vi "S2C_SaveScriptAs.vi"(8 "Error In":errorcluster) -> (0 "Error Out":errorcluster)   [LabVIEW 2015]
doc: "Prompts for file name, checks the script settings, and saves the script to a local file."
uses:
  Globals/S2C_Globals.vi
  <vilib>/Utility/config.llb/Write Key (String).vi
  <vilib>/Utility/config.llb/NI_LVConfig.lvlib
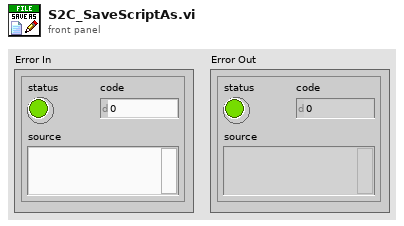
[diagram p1: front panel]
types:
  T1 = typedef "NI_LVConfig.lvlib/Config Data RefNum.ctl" = refnum<k1>
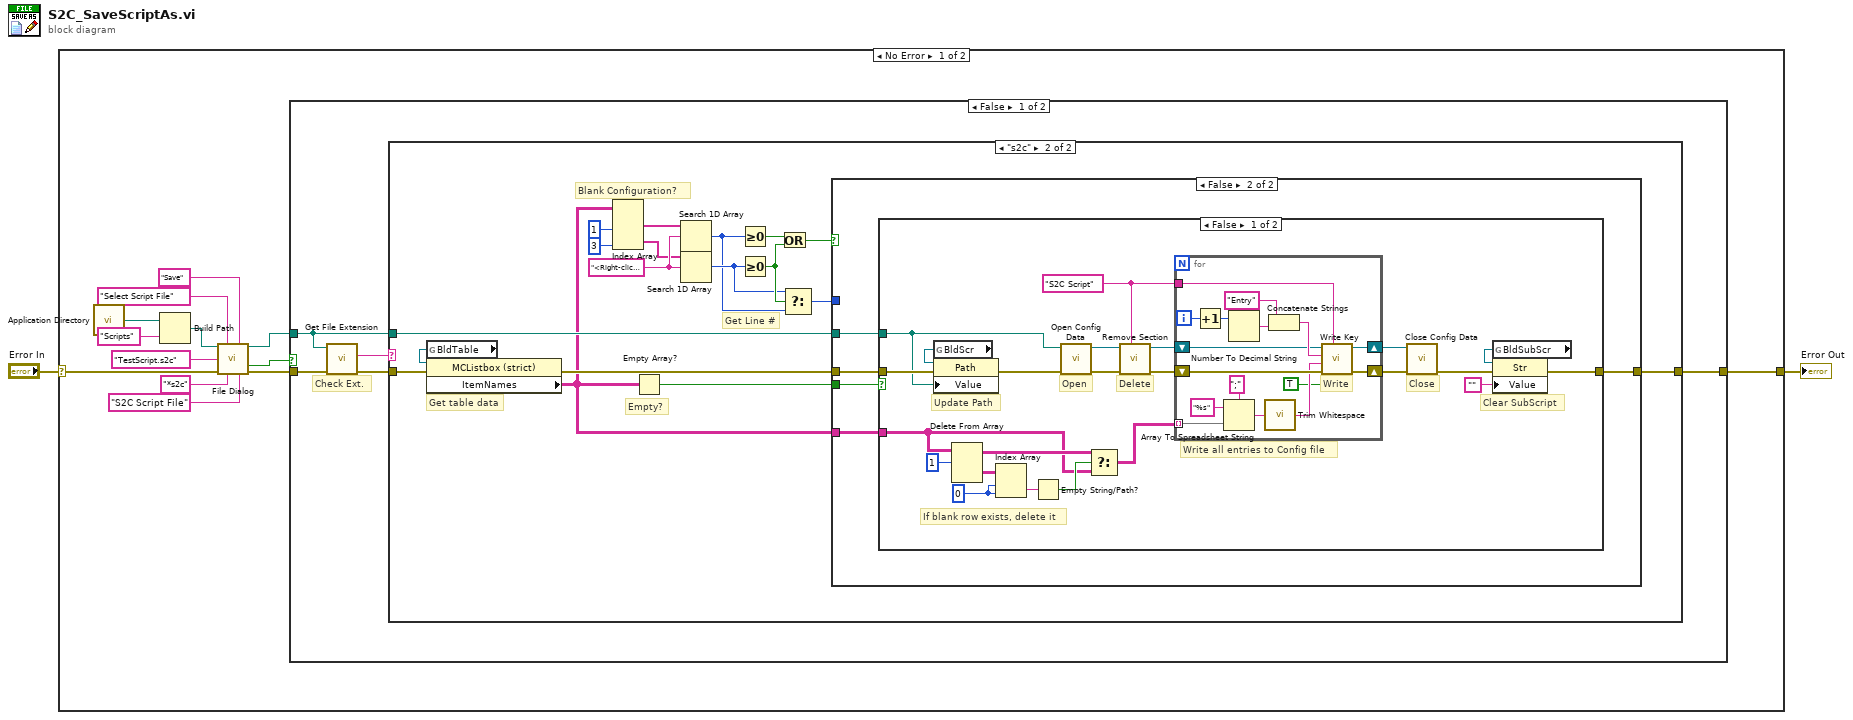
[diagram p0: block diagram]
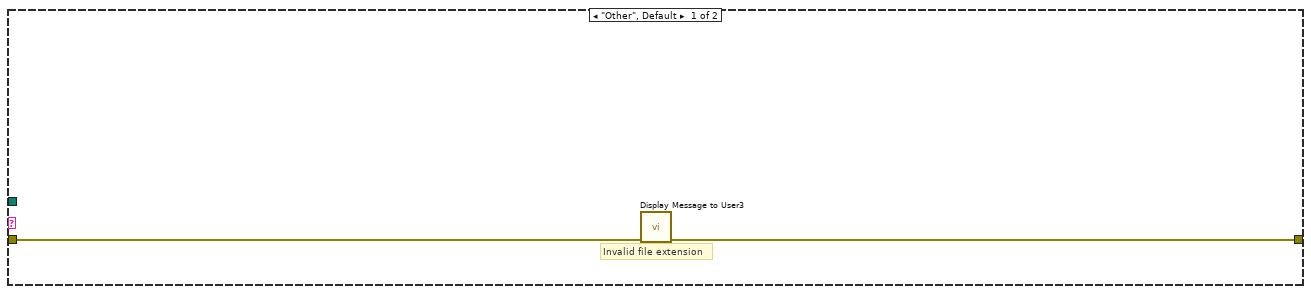
[diagram p2: hidden frame]
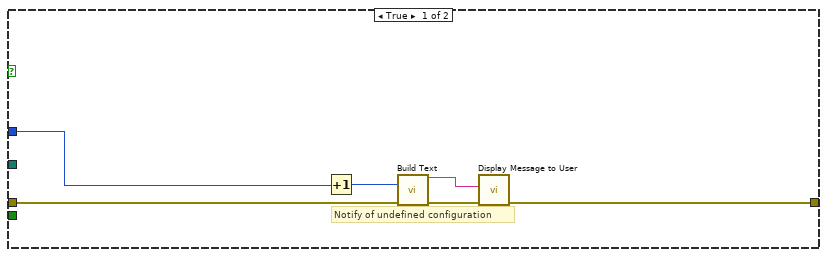
[diagram p3: hidden frame]
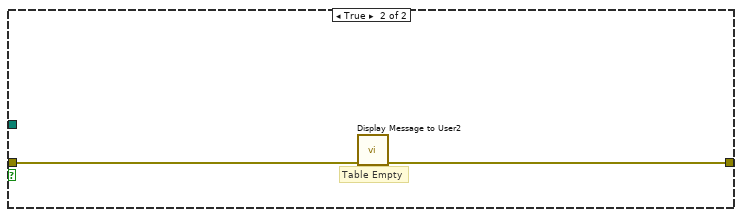
[diagram p4: hidden frame]
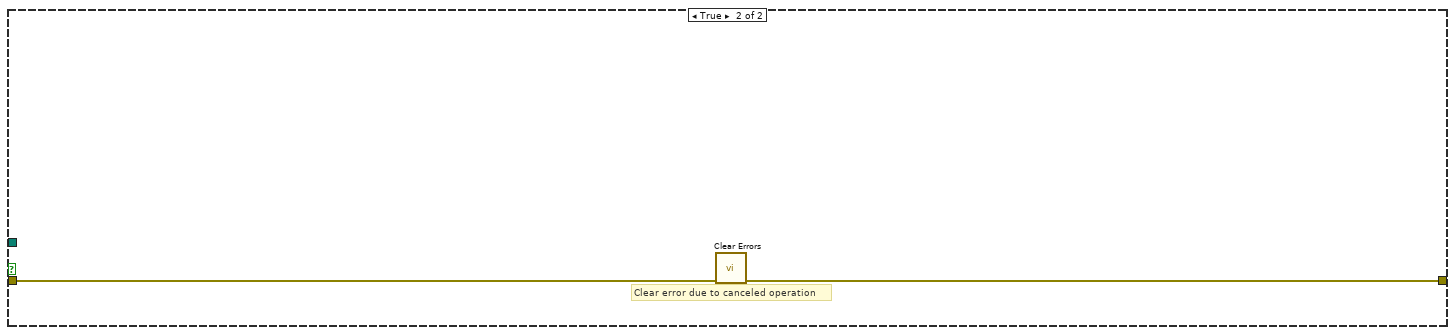
[diagram p5: hidden frame]
diagram:
  n1 = case shown="No Error" "Error In" {
    selector: "Error In" -> [w15 w95]
    tunnel: [w3 w95] -> w1
    frame No Error {
      n2 = call <vilib>:"Application Directory.vi"() -> ("Application Directory"=w13:path)
      n3 = Build Path(base path=w13, name or relative path="Scripts") -> (appended path=w11:path)
      n4 = call "File Dialog"("start path"=w11, "prompt"="Select Script File", "button label"="Save", "default name"="TestScript.s2c", "error in"=w15, "pattern (all files)"="*s2c", "pattern label"="S2C Script File") -> ("selected path"=w4:path, "cancelled"=w5:bool, "error out"=w6:errorcluster)  [unwired: 5 in, 1 out]
      n5 = case shown="False" w5 {
        tunnel: w6 -> [w19 w94]
        tunnel: w4 -> [w16 _]
        tunnel: [w20 w93] -> w3
        frame False {
          # "Check Ext."
          n6 = call <vilib>:"Get File Extension.vi"("error in (no error)"=w19, "file"=w16) -> ("error out"=w18:errorcluster, "lowercase file extension"=w17:string)  [unwired: 5 in, 3 out]
          n7 = case shown="\"s2c\"" w17 {
            tunnel: [w21 w39] -> w20
            tunnel: w18 -> [w22 w37]
            tunnel: w16 -> [_ w36]
            frame "Other", Default {
              # "Invalid file extension"
              n8 = call "Display Message to User3"("error in (no error)"=w22) -> ("error out"=w21:errorcluster)  [unwired: 9 in, 1 out]
            }
            frame "s2c" {
              w31 = "<Right-click to configure>"
              # "Get Line #"
              # "Blank Configuration?"
              # "Get table data"
              # "Empty?"
              n9 = global read "S2C_Globals.vi" "BldTable"() -> (w38:refnum<vi>)
              n10 = property class="MCListbox (strict)"(reference=w38, error in=w37) -> (error out=w40:errorcluster, "ItemNames"=w34:string[][])  [unwired: 1 out]
              n11 = Index Array(array=w34, index (col) #1=1 ("disabled index (col)"), index (col) #2=3 ("index (col)")) -> (element #1=w32:string[], element #2=w29:string[])  [unwired: 2 in]
              n12 = Empty Array?(array=w34) -> (empty?=w33:bool)
              n13 = Search 1D Array(1D array=w32, element=w31) -> (index of element=w24:i32)  [unwired: 1 in]
              n14 = Search 1D Array(1D array=w29, element=w31) -> (index of element=w25:i32)  [unwired: 1 in]
              n15 = Greater Or Equal To 0?(x=w24) -> (x >= 0?=w28:bool)
              n16 = Greater Or Equal To 0?(x=w25) -> (x >= 0?=w26:bool)
              n17 = Or(x=w28, y=w26) -> (x .or. y?=w27:bool)
              n18 = Select(t=w25, s=w26, f=w24) -> (s? t:f=w23:i32)
              n19 = case shown="False" w27 {
                tunnel: w40 -> [w46 w51]
                tunnel: [w43 w50] -> w39
                tunnel: w36 -> [_ w48]
                tunnel: w34 -> [_ w49]
                tunnel: w33 -> [_ w47]
                tunnel: w23 -> [w41 _]
                frame True {
                  # "Notify of undefined configuration"
                  n20 = Increment(x=w41) -> (x+1=w42:i32)
                  n21 = call "Build Text"("Line"=w42, "error in (no error)"=w46) -> ("Result"=w44:string, "error out"=w45:errorcluster)  [unwired: 12 in]
                  n22 = call "Display Message to User"("error in (no error)"=w45, "Message"=w44) -> ("error out"=w43:errorcluster)  [unwired: 8 in, 1 out]
                }
                frame False {
                  n23 = case shown="False" w47 {
                    tunnel: w51 -> [w58 w92]
                    tunnel: [w52 w91] -> w50
                    tunnel: w49 -> [w60 _]
                    tunnel: w48 -> [w56 _]
                    frame False {
                      w67 = 0 ("index (row)")
                      w61 = "S2C Script"
                      # "Clear SubScript"
                      # "Update Path"
                      # "Write all entries to Config file"
                      # "If blank row exists, delete it"
                      # "Delete"
                      # "Close"
                      # "Open"
                      n24 = global read "S2C_Globals.vi" "BldScr"() -> (w59:refnum<vi>)
                      n25 = property class="Path"(reference=w59, error in=w58, "Value"=w56) -> (error out=w57:errorcluster)  [unwired: 1 out]
                      n26 = Delete From Array(array=w60, length=1) -> (deleted portion=w68:string[][], array with subset deleted=w70:string[][])  [unwired: 2 in]
                      n27 = Index Array(array=w68, index (row)=w67, index (col)=w67) -> (element=w66:string)
                      n28 = Empty String/Path?(string/path=w66) -> (empty?=w65:bool)
                      n29 = call <vilib>:"Open Config Data.vi"("error in (no error)"=w57, "configuration file path"=w56) -> ("error out"=w74:errorcluster, "refnum"=w63:T1)  [unwired: 7 in, 1 out]
                      n30 = Select(t=w70, s=w65, f=w60) -> (s? t:f=w69:string[][])
                      n31 = call <vilib>:"Remove Section.vi"("section"=w61, "error in (no error)"=w74, "refnum"=w63) -> ("error out"=w64:errorcluster, "refnum out"=w62:T1)  [unwired: 6 in, 1 out]
                      n32 = for {
                        tunnel: w69 -> [w90] mode=indexing
                        shift-right: [w82] -> w73
                        shift-left: w64 -> [w83]
                        tunnel: w61 -> [w79]
                        shift-right: [w77] -> w72
                        shift-left: w62 -> [w78]
                        i -> [w88]
                        # "Write"
                        n33 = Increment(x=w88) -> (x+1=w87:i32)
                        n34 = Array To Spreadsheet String(delimiter (Tab)=";", array=w90, 3:"%s" ("format string")) -> (spreadsheet string=w81:string)
                        n35 = Number To Decimal String(number=w87) -> (decimal integer string=w85:string)  [unwired: 1 in]
                        n36 = call <vilib>:"Trim Whitespace.vi"("string"=w81) -> ("trimmed string"=w76:string)  [unwired: 1 in]
                        n37 = Concatenate Strings("Entry" ("string"), w85) -> (w80:string)
                        n38 = call-poly <vilib>:"Write Key.vi"("write raw string? (F)"=TRUE, "section"=w79, "error in (no error)"=w83, "value"=w76, "key"=w80, "refnum"=w78) -> ("error out"=w82:errorcluster, "refnum out"=w77:T1)  [unwired: 3 in, 1 out]
                      }
                      n39 = call <vilib>:"Close Config Data.vi"("error in (no error)"=w73, "refnum"=w72) -> ("error out"=w54:errorcluster)  [unwired: 8 in, 1 out]
                      n40 = global read "S2C_Globals.vi" "BldSubScr"() -> (w55:refnum<vi>)
                      n41 = property class="Str"(reference=w55, error in=w54, "Value"="") -> (error out=w52:errorcluster)  [unwired: 1 out]
                    }
                    frame True {
                      # "Table Empty"
                      n42 = call "Display Message to User2"("error in (no error)"=w92) -> ("error out"=w91:errorcluster)  [unwired: 9 in, 1 out]
                    }
                  }
                }
              }
            }
          }
        }
        frame True {
          # "Clear error due to canceled operation"
          n43 = call <vilib>:"Clear Errors.vi"("error in (no error)"=w94) -> ("error out"=w93:errorcluster)  [unwired: 5 in, 1 out]
        }
      }
    }
    frame Error {
    }
  }
  "Error Out" <- w1
